vi "module connect Through Link Module.vi"(8 "error in (no error)":errorcluster, 9 "result":cluster{"value":i32, "error":i32}, 10 "id_linkStem":u32, 11 "id":u32) -> (0 "error out":errorcluster, 1 "result out":cluster{"value":i32, "error":i32}, 2 "id_linkStem out":u32, 3 "id out":u32)   [LabVIEW 2021, in "BrainStem2_LabVIEW_Library.lvlib"]
doc: "aLIBEXPORT void __stdcall module_connectThroughLinkModule(unsigned int* id, unsigned int* id_linkStem, struct Result* result);"
uses:
  BrainStem2_LabVIEW_Library.lvlib
  BrainStem2_LabVIEW.dll
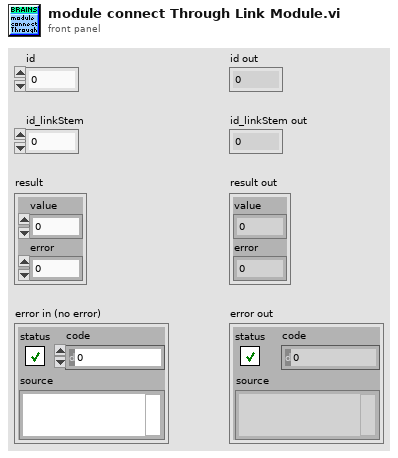
[diagram p1: front panel]
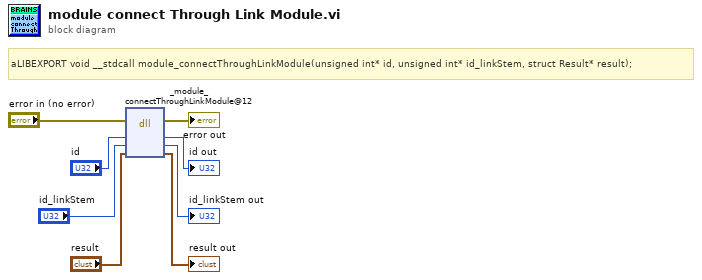
[diagram p0: block diagram]
diagram:
  # "aLIBEXPORT void __stdcall module_connectThroughLinkModule(unsigned int* id, unsigned int* id_linkStem, struct Result* result);"
  n1 = dll-call lib="C:/DEV-TDS/Canary/T20029/T20029-80004 BS2 PROG SW/src/drivers/acroname/development/LabVIEW/BrainStem2_LabVIEW_w32/BrainStem2_LabVIEW_w32/BrainStem2_LabVIEW.*" fn="_module_connectThroughLinkModule@12"(error in="error in (no error)", "id"="id", "id_linkStem"="id_linkStem", "result"="result") -> (error out=→"error out":errorcluster, "id"=→"id out":u32, "id_linkStem"=→"id_linkStem out":u32, "result"=→"result out":cluster{"value":i32, "error":i32})  [unwired: 3 in, 1 out]
